vi "GEvt-Filter Global Log - v1.0.vi"(7 "Rules-v1":T1, 8 "Matched Previous?":bool, 11 "Cross CSM Data (In)":T4) -> (0 "Matched? (Dup)":bool, 3 "Cross CSM Data":T4)   [LabVIEW 2017, in "Communicable State Machine.lvlib"]
doc: "### GEvt-Filter Global Log - v1.0.vi\n\n-- <b>Controls</b> --\n- <b>Rules-v1</b>:\n- <b>Cross CSM Data (in)</b>:\n\n-- <b>Indicators</b> --\n- <b>Matched? (dup)</b>:\n- <b>Cross CSM Data</b>:"
uses:
  Communicable State Machine.lvlib
  Typedef/_CSM_GlobalLog_MSG.ctl
  Typedef/_CSM_Response Source Message.ctl
  Typedef/_CSM_GlobalLog_MSG_TYPE.ctl
  Typedef/_CSM_GlobalLog Filter Rules - v1.0.ctl
  Typedef/_CSM_GlobalLog_STATE_TYPE.ctl
  LogFilter/SettingVIs/Set CSM StateType Filter.vi
  LogFilter/SettingVIs/Set Global StateType Filter.vi
  LogFilter/SettingVIs/Set CSM State Filter.vi
  LogFilter/SettingVIs/Set CSM LogType Filter.vi
  LogFilter/SettingVIs/Set Global State Filter.vi
  LogFilter/SettingVIs/Set Global LogType Filter.vi
  LogFilter/SettingVIs/Set Global CSM Filter.vi
  LogFilter/LogFilter.lvclass
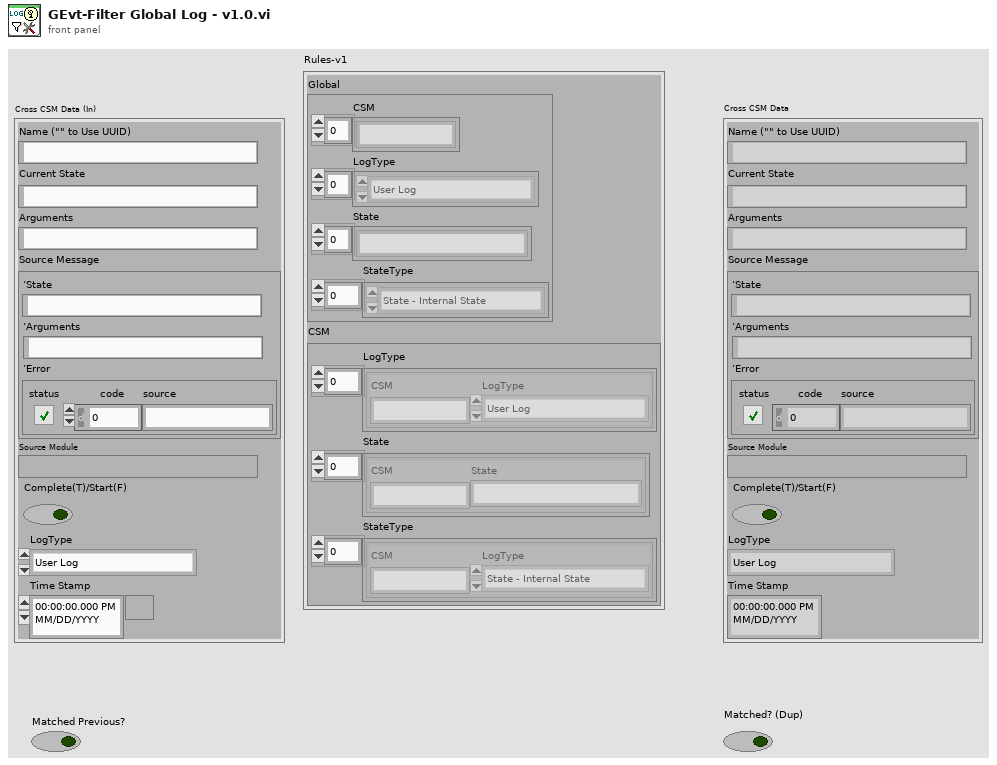
[diagram p1: front panel]
types:
  T1 = typedef "Communicable State Machine.lvlib/_CSM_GlobalLog Filter Rules - v1.0.ctl" = cluster{"Global":cluster{"CSM":string[], "LogType":T2[], "State":string[], "StateType":T3[]}, "CSM":cluster{"LogType":cluster{"CSM":string, "LogType":T2}[], "State":cluster{"CSM":string, "State":string}[], "StateType":cluster{"CSM":string, "LogType":T3}[]}}
  T2 = typedef "Communicable State Machine.lvlib/_CSM_GlobalLog_MSG_TYPE.ctl" = enum16{"User Log", "State Change", "Status", "Interrupt", "Register", "Unregister", "Error Log", "Module Created", "Module Destroyed", "Async Message", "No-Rep Async Message", "Sync Message", "AsyncMsg Complete", "SyncMsg Complete"}
  T3 = typedef "Communicable State Machine.lvlib/_CSM_GlobalLog_STATE_TYPE.ctl" = enum16{"State - Internal State", "State - External Message", "State - Response", "State - Complete"}
  T4 = typedef "Communicable State Machine.lvlib/_CSM_GlobalLog_MSG.ctl" = cluster{"Name (\"\" to Use UUID)":string, "Current State":string, "Arguments":string, "Source Message":T5, "Source Module":string, "Complete(T)/Start(F)":bool, "LogType":T2, "Time Stamp":timestamp}
  T5 = typedef "Communicable State Machine.lvlib/_CSM_Response Source Message.ctl" = cluster{"‘State":string, "’Arguments":string, "’Error":errorcluster}
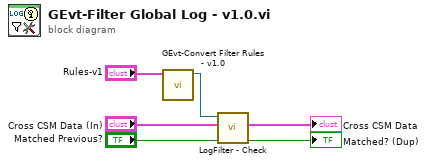
[diagram p0: block diagram]
diagram:
  n1 = call "GEvt-Convert Filter Rules - v1.0.vi"("Rules-v1"="Rules-v1") -> ("GlobalLogFilter"=w2:refnum<class "LogFilter.lvclass">)  [unwired: 10 in]
  n2 = call "LogFilter - Check.vi"("Matched Previous?"="Matched Previous?", "Cross CSM Data In"="Cross CSM Data (In)", "GlobalLogFilter In"=w2) -> ("Matched? (Dup)"=→"Matched? (Dup)":bool, "Cross CSM Data Out"=→"Cross CSM Data":T4)  [unwired: 6 in, 1 out]
